vi "speed culculation 1.2.vi"(8 "i":i32, 9 "Speed(RPM)":dbl, 10 "distance":dbl, 11 "dt(s)":dbl) -> (0 "complet?":bool, 1 "t2?":bool, 3 "Speed":dbl, 4 "t2":dbl)   [LabVIEW 2019]
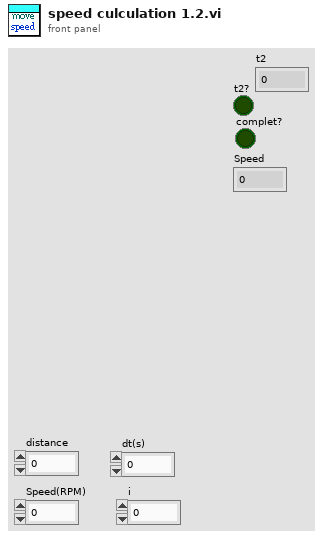
[diagram p1: front panel]
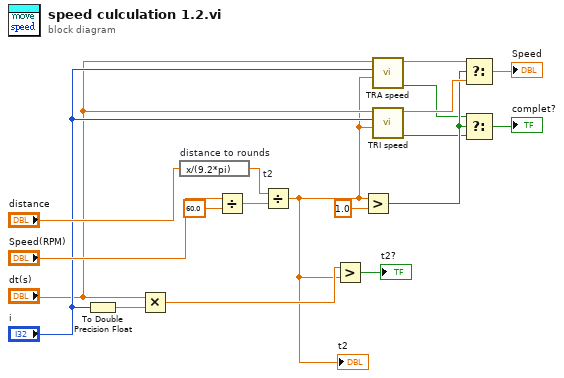
[diagram p0: block diagram]
diagram:
  n1 = To Double Precision Float(number="i") -> (double precision float=w14:dbl)
  n2 = Multiply(x="dt(s)", y=w14) -> (x*y=w11:dbl)
  n3 = expression code="x/(9.2*pi)" "distance to rounds"("distance") -> (w16:dbl)
  n4 = Divide(x="Speed(RPM)", y=60.0) -> (x/y=w15:dbl)
  n5 = Divide "t2"(x=w16, y=w15) -> (x/y=w9:dbl)
  "t2" <- w9
  n6 = Greater?(x=w11, y=w9) -> (0:→"t2?":bool)
  n7 = Greater?(x=w9, y=1.0) -> (0:w5:bool)
  n8 = call "TRA speed.vi"("t2"=w9, "i"="i", "dt(s)"="dt(s)") -> ("complet?"=w4:bool, "Waveform Chart"=w7:dbl)  [unwired: 7 in]
  n9 = call "TRI speed.vi"("t2"=w9, "i"="i", "dt(s)"="dt(s)") -> ("complet?"=w3:bool, "Waveform Chart"=w6:dbl)  [unwired: 7 in]
  n10 = Select(t=w7, s=w5, f=w6) -> (s? t:f=→"Speed":dbl)
  n11 = Select(t=w4, s=w5, f=w3) -> (s? t:f=→"complet?":bool)
